vi "frame counter.vi"(8 "stop ref":refnum<vi>, 11 "frame count ref":refnum<vi>) -> ()   [LabVIEW 2017]
uses:
  <vilib>/Platform/TimedLoop/XDataNode/timing_clust.ctl
  <vilib>/Platform/TimedLoop/XDataNode/nitl_modes.ctl
  <vilib>/Platform/TimedLoop/XDataNode/wakeup.ctl
  <vilib>/DAQmx/read.llb/DAQmx Read (Counter U32 1Chan 1Samp).vi
  PushTask Globals.vi
  <vilib>/DAQmx/miscellaneous.llb/DAQmx Fill In Error Info.vi
  <vilib>/platform/TimedLoop/XDataNode/XDataNode.xnode
  <vilib>/Platform/TimedLoop/XDataNode/XDNodeRunTimeDep.lvlib
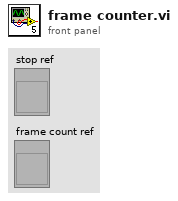
[diagram p1: front panel]
types:
  T1 = typedef "XDNodeRunTimeDep.lvlib/timing_clust.ctl" = cluster{"Expected End [f-1]":u64, "Actual End [f-1]":u64, "Finished Late? [f-1]":bool, "Expected End [i-1]":u64, "Actual End [i-1]":u64, "Finished Late? [i-1]":bool, "Expected Start [i]":u64, "Actual Start [i]":u64, "Expected Start [f]":u64, "Actual Start [f]":u64, "Source Name":string, "Structure Name":string, "Period":i64, "Deadline":i64, "Offset":i64, "Start":i64, "Priority":i32, "Timeout":i32, "Mode":T2, "Wakeup Reason":T3, "Error":errorcluster, "Source Type":string, "Secondary Source Type":string, "Global End Time":u64, "Global Start Time":u64, "Frame Duration":u64, "Iteration Duration":u64, "Assigned CPU":i32, "I/O Scan Engine Mode":u32}
  T2 = typedef "XDNodeRunTimeDep.lvlib/nitl_modes.ctl" = enum32{"No Change", "Process missed periods, maintain original phase", "Discard missed periods, maintain original phase", "Process missed periods, ignore original phase", "Discard missed periods, ignore original phase"}
  T3 = typedef "XDNodeRunTimeDep.lvlib/wakeup.ctl" = enum32{"Normal", "Aborted", "Asynchronous wakeup", "Timing source error", "Timed loop error", "Timeout"}
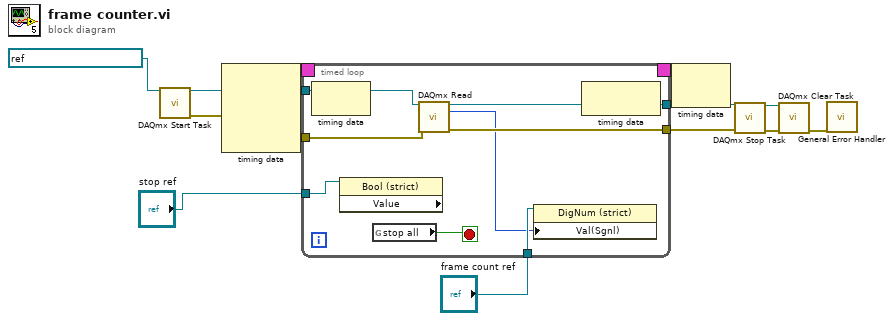
[diagram p0: block diagram]
diagram:
  n1 = call <vilib>:"DAQmx Start Task.vi"("task/channels in"=refnum<k21> "frame counter_Dev1") -> ("task out"=w12:refnum<k21>, "error out"=w9:errorcluster)  [unwired: 13 in]
  n2 = node-c288() -> (w3:T1)  [unwired: 4 in]
  n3 = timed-loop {
    tunnel: w12 -> [w20]
    tunnel: w9 -> [w19]
    tunnel: [w18] -> w8
    tunnel: [w17] -> w7
    tunnel: "frame count ref" -> [w16]
    tunnel: "stop ref" -> [w15]
    timing: w3 -> [_]
    timing-out: [_] -> w2
    stop <- w13 stop-if-true
    n4 = node-c288() -> ()  [unwired: 1 in, 1 out]
    n5 = property class="Bool (strict)" props=["Value"](reference=w15) -> ()  [unwired: 1 in, 3 out]
    n6 = global read "PushTask Globals.vi" "stop all"() -> (w13:bool)
    n7 = call-poly <vilib>:"DAQmx Read.vi"("task/channels in"=w20, "error in"=w19) -> ("task out"=w18:refnum<k21>, "data"=w14:u32, "error out"=w17:errorcluster)  [unwired: 11 in]
    n8 = property class="DigNum (strict)"(reference=w16, "Val(Sgnl)"=w14) -> ()  [unwired: 1 in, 2 out]
    n9 = node-c288() -> ()  [unwired: 1 in, 1 out]
  }
  n10 = node-c288(w2) -> ()  [unwired: 1 out]
  n11 = call <vilib>:"DAQmx Stop Task.vi"("task/channels in"=w8, "error in"=w7) -> ("task out"=w11:refnum<k21>, "error out"=w10:errorcluster)  [unwired: 12 in]
  n12 = call <vilib>:"DAQmx Clear Task.vi"("task in"=w11, "error in"=w10) -> ("error out"=w4:errorcluster)  [unwired: 13 in]
  n13 = call <vilib>:"General Error Handler.vi"("error in (no error)"=w4) -> ()  [unwired: 10 in, 5 out]
